vi "Handle_Plot.vi"(2 "Graph reference":refnum<vi>[](array[refnum]), 3 "System Monitor Variables (in)":T2={"Time"=[], "LI1CH1"=[], "LI1CH2"=[], "LI2CH1"=[], "LI2CH2"=[], "LI3CH1"=[], "LI3CH2"=[], "Field"=[], "Temp"=[], "Temp 2"=[], "Temp 3"=[], "N_Level"=[], "H_Level"=[], "Heat_370"=[], "Sorb_Heat"=[], "Still_Heat"=[], "Capacity"=[], "Loss"=[], "Magnet_Temperature"=[], "Lam_Pressure"=[], "Lam_NValve"=[], "370-T1"=[], "370-T2"=[], "370-T3"=[], "370-T4"=[], "370-T5"=[], "370-R1"=[], "370-R2"=[], "370-R3"=[], "370-R4"=[], "370-R5"=[], "372-T1"=[], "372-T2"=[], "372-T3"=[], "372-T4"=[], "372-T5"=[], "372-T6"=[], "372-R1"=[], "372-R2"=[], "372-R3"=[], "372-R4"=[], "372-R5"=[], "372-R6"=[], "Nada"=[nan], "K2440_Res"=[], "K2440_Current"=[], "VTI_Heater"=[], "VTI_NValve"=[], "LS340_Heater"=[], "K6221_Amplitude"=[], "K6221_Frequency"=[], "Cond_Pressure"=[], "Still_Pressure"=[], "FP_Out_Pressure"=[], "Dump_Pressure"=[], "V1"=[], "V2"=[], "V4"=[], "V5"=[], "V9"=[], "Forepump"=[], "Compressor"=[], "K6221_Offset"=[], "BoxTemp"=[], "By"=[], "Bz"=[], "Phi"=[], "heater-recond (%)"=[], "Dewar Pressure "=[], "JT-SP-Control"=[], "350 T1"=[], "350 T2"=[], "350 T3"=[], "350 T4"=[], "350 R1"=[], "350 R2"=[], "350 R3"=[], "350 R4"=[], "Angle"=[]}, 4 "Plot Array (in)":T1[](array[typedef]) {"Y-Axis Array" items=["Time", "LI1CH1", "LI1CH2", "LI2CH1", "LI2CH2", "LI3CH1", "LI3CH2", "Field", "Temp", "Temp 2", "Temp 3", "N_Level", "H_Level", "Heat_370", "Sorb_Heat", "Still_Heat", "Capacity", "Loss", "Magnet_Temperature", "Lam_Pressure", "Lam_NValve", "370-T1", "370-T2", "370-T3", "370-T4", "370-T5", "370-R1", "370-R2", "370-R3", "370-R4", "370-R5", "372-T1", "372-T2", "372-T3", "372-T4", "372-T5", "372-T6", "372-R1", "372-R2", "372-R3", "372-R4", "372-R5", "372-R6", "Nada", "K2440_Res", "K2440_Current", "VTI_Heater", "VTI_NValve", "LS340_Heater", "K6221_Amplitude", "K6221_Frequency", "Cond_Pressure", "Still_Pressure", "FP_Out_Pressure", "Dump_Pressure", "V1", "V2", "V4", "V5", "V9", "Forepump", "Compressor", "K6221_Offset", "BoxTemp", "By", "Bz", "Phi", "heater-recond (%)", "Dewar Pressure ", "JT-SP-Control", "350 T1", "350 T2", "350 T3", "350 T4", "350 R1", "350 R2", "350 R3", "350 R4", "Angle"]; "X-Axis" items=["Time", "LI1CH1", "LI1CH2", "LI2CH1", "LI2CH2", "LI3CH1", "LI3CH2", "Field", "Temp", "Temp 2", "Temp 3", "N_Level", "H_Level", "Heat_370", "Sorb_Heat", "Still_Heat", "Capacity", "Loss", "Magnet_Temperature", "Lam_Pressure", "Lam_NValve", "370-T1", "370-T2", "370-T3", "370-T4", "370-T5", "370-R1", "370-R2", "370-R3", "370-R4", "370-R5", "372-T1", "372-T2", "372-T3", "372-T4", "372-T5", "372-T6", "372-R1", "372-R2", "372-R3", "372-R4", "372-R5", "372-R6", "Nada", "K2440_Res", "K2440_Current", "VTI_Heater", "VTI_NValve", "LS340_Heater", "K6221_Amplitude", "K6221_Frequency", "Cond_Pressure", "Still_Pressure", "FP_Out_Pressure", "Dump_Pressure", "V1", "V2", "V4", "V5", "V9", "Forepump", "Compressor", "K6221_Offset", "BoxTemp", "By", "Bz", "Phi", "heater-recond (%)", "Dewar Pressure ", "JT-SP-Control", "350 T1", "350 T2", "350 T3", "350 T4", "350 R1", "350 R2", "350 R3", "350 R4", "Angle"]}) -> (1 "Measurement Graphs":T1[](array[typedef]) {"Y-Axis Array" items=["Time", "LI1CH1", "LI1CH2", "LI2CH1", "LI2CH2", "LI3CH1", "LI3CH2", "Field", "Temp", "Temp 2", "Temp 3", "N_Level", "H_Level", "Heat_370", "Sorb_Heat", "Still_Heat", "Capacity", "Loss", "Magnet_Temperature", "Lam_Pressure", "Lam_NValve", "370-T1", "370-T2", "370-T3", "370-T4", "370-T5", "370-R1", "370-R2", "370-R3", "370-R4", "370-R5", "372-T1", "372-T2", "372-T3", "372-T4", "372-T5", "372-T6", "372-R1", "372-R2", "372-R3", "372-R4", "372-R5", "372-R6", "Nada", "K2440_Res", "K2440_Current", "VTI_Heater", "VTI_NValve", "LS340_Heater", "K6221_Amplitude", "K6221_Frequency", "Cond_Pressure", "Still_Pressure", "FP_Out_Pressure", "Dump_Pressure", "V1", "V2", "V4", "V5", "V9", "Forepump", "Compressor", "K6221_Offset", "BoxTemp", "By", "Bz", "Phi", "heater-recond (%)", "Dewar Pressure ", "JT-SP-Control", "350 T1", "350 T2", "350 T3", "350 T4", "350 R1", "350 R2", "350 R3", "350 R4", "Angle"]; "X-Axis" items=["Time", "LI1CH1", "LI1CH2", "LI2CH1", "LI2CH2", "LI3CH1", "LI3CH2", "Field", "Temp", "Temp 2", "Temp 3", "N_Level", "H_Level", "Heat_370", "Sorb_Heat", "Still_Heat", "Capacity", "Loss", "Magnet_Temperature", "Lam_Pressure", "Lam_NValve", "370-T1", "370-T2", "370-T3", "370-T4", "370-T5", "370-R1", "370-R2", "370-R3", "370-R4", "370-R5", "372-T1", "372-T2", "372-T3", "372-T4", "372-T5", "372-T6", "372-R1", "372-R2", "372-R3", "372-R4", "372-R5", "372-R6", "Nada", "K2440_Res", "K2440_Current", "VTI_Heater", "VTI_NValve", "LS340_Heater", "K6221_Amplitude", "K6221_Frequency", "Cond_Pressure", "Still_Pressure", "FP_Out_Pressure", "Dump_Pressure", "V1", "V2", "V4", "V5", "V9", "Forepump", "Compressor", "K6221_Offset", "BoxTemp", "By", "Bz", "Phi", "heater-recond (%)", "Dewar Pressure ", "JT-SP-Control", "350 T1", "350 T2", "350 T3", "350 T4", "350 R1", "350 R2", "350 R3", "350 R4", "Angle"]})   [LabVIEW 2016]
uses:
  Global/Global Variables/System Monitor Cluster.ctl
  Plot.ctl
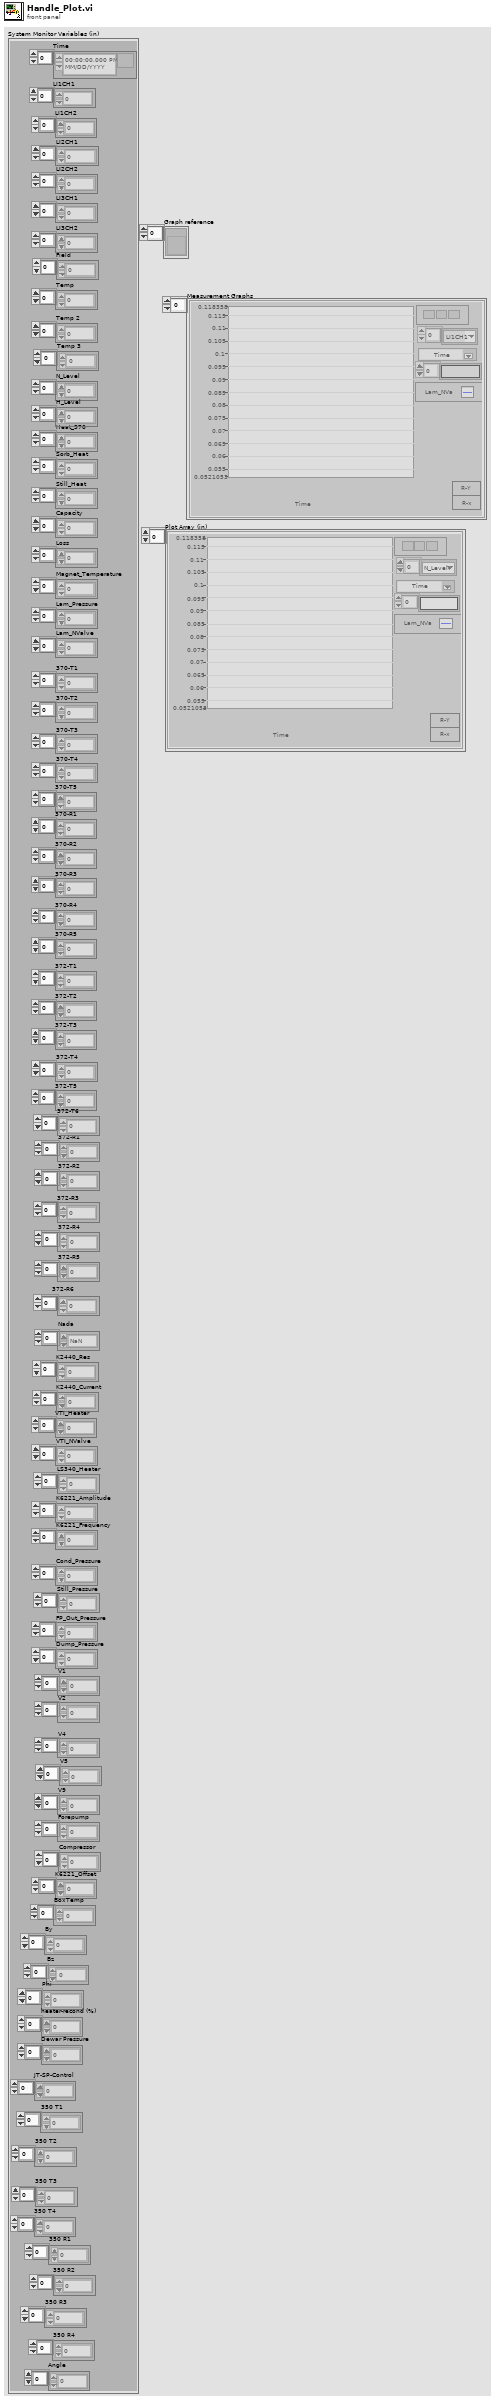
[diagram p1: front panel]
types:
  T1 = typedef "Plot.ctl" = cluster{"Measurement Graph":cluster{"Y":dbl[], "X":dbl[]}[], "X-Axis":i16, "Y-Axis Array":i16[], "Scale Plot":string[], "Rescale X":bool, "Rescale Y":bool}
  T2 = typedef "System Monitor Cluster.ctl" = cluster{"Time":timestamp[], "LI1CH1":dbl[], "LI1CH2":dbl[], "LI2CH1":dbl[], "LI2CH2":dbl[], "LI3CH1":dbl[], "LI3CH2":dbl[], "Field":dbl[], "Temp":dbl[], "Temp 2":dbl[], "Temp 3":dbl[], "N_Level":dbl[], "H_Level":dbl[], "Heat_370":dbl[], "Sorb_Heat":dbl[], "Still_Heat":dbl[], "Capacity":dbl[], "Loss":dbl[], "Magnet_Temperature":dbl[], "Lam_Pressure":dbl[], "Lam_NValve":dbl[], "370-T1":dbl[], "370-T2":dbl[], "370-T3":dbl[], "370-T4":dbl[], "370-T5":dbl[], "370-R1":dbl[], "370-R2":dbl[], "370-R3":dbl[], "370-R4":dbl[], "370-R5":dbl[], "372-T1":dbl[], "372-T2":dbl[], "372-T3":dbl[], "372-T4":dbl[], "372-T5":dbl[], "372-T6":dbl[], "372-R1":dbl[], "372-R2":dbl[], "372-R3":dbl[], "372-R4":dbl[], "372-R5":dbl[], "372-R6":dbl[], "Nada":dbl[], "K2440_Res":dbl[], "K2440_Current":dbl[], "VTI_Heater":dbl[], "VTI_NValve":dbl[], "LS340_Heater":dbl[], "K6221_Amplitude":dbl[], "K6221_Frequency":dbl[], "Cond_Pressure":dbl[], "Still_Pressure":dbl[], "FP_Out_Pressure":dbl[], "Dump_Pressure":dbl[], "V1":dbl[], "V2":dbl[], "V4":dbl[], "V5":dbl[], "V9":dbl[], "Forepump":dbl[], "Compressor":dbl[], "K6221_Offset":dbl[], "BoxTemp":dbl[], "By":dbl[], "Bz":dbl[], "Phi":dbl[], "heater-recond (%)":dbl[], "Dewar Pressure ":dbl[], "JT-SP-Control":dbl[], "350 T1":dbl[], "350 T2":dbl[], "350 T3":dbl[], "350 T4":dbl[], "350 R1":dbl[], "350 R2":dbl[], "350 R3":dbl[], "350 R4":dbl[], "Angle":dbl[]}
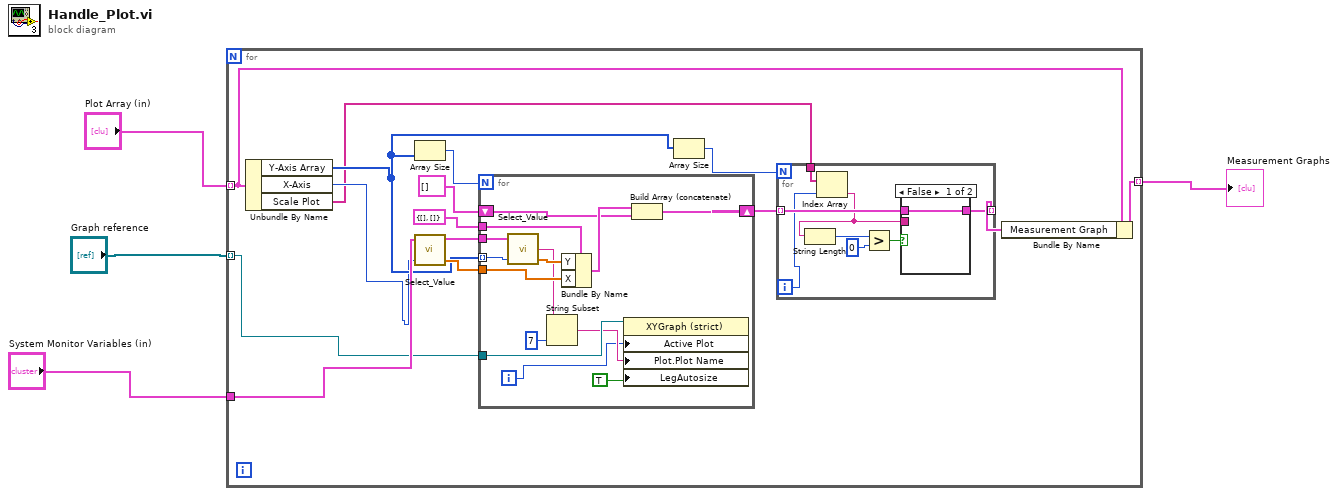
[diagram p0: block diagram]
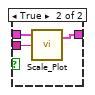
[diagram p2: hidden frame]
diagram:
  n1 = for {
    tunnel: "System Monitor Variables (in)" -> [w13]
    tunnel: [w7] -> w2 mode=indexing
    tunnel: "Plot Array (in)" -> [w9] mode=indexing
    tunnel: "Graph reference" -> [w5] mode=indexing
    n2 = Unbundle By Name(w9) -> ("Y-Axis Array"=w11:i16[], "X-Axis"=w10:i16, "Scale Plot"=w6:string[])
    n3 = Array Size(array=w11) -> (size(s)=w12:i32)
    n4 = call "Select_Value.vi"("Numerisch"=w10, "System Monitor Variables"=w13) -> ("Array"=w16:dbl[])  [unwired: 1 in, 2 out]
    n5 = for {
      N: w12 -> [_]
      tunnel: cluster{"X":dbl[], "Y":dbl[]} {"X"=[], "Y"=[]} -> [w44]
      tunnel: w11 -> [w42] mode=indexing
      tunnel: w13 -> [w41]
      shift-right: [w40] -> w14
      shift-left: cluster{"X":dbl[], "Y":dbl[]}[] [] -> [w33]
      tunnel: w16 -> [w39]
      tunnel: w5 -> [w36]
      i -> [w31]
      n6 = call "Select_Value.vi"("Numerisch"=w42, "System Monitor Variables"=w41) -> ("Array"=w43:dbl[], "String"=w37:string)  [unwired: 1 in, 1 out]
      n7 = String Subset(string=w37, length (rest)=7 ("length (rest)")) -> (substring=w32:string)  [unwired: 1 in]
      n8 = Bundle By Name(cluster=w44, "Y"=w43, "X"=w39) -> (w34:cluster{"X":dbl[], "Y":dbl[]})
      n9 = property on="Property Node" class="XYGraph (strict)"(reference=w36, "Active Plot"=w31, "Plot.Plot Name"=w32, "LegAutosize"=TRUE) -> ()  [unwired: 1 in, 2 out]
      n10 = Build Array (concatenate)(w34, w33) -> (w40:cluster{"X":dbl[], "Y":dbl[]}[])
    }
    n11 = Array Size(array=w11) -> (size(s)=w15:i32)
    n12 = for {
      N: w15 -> [_]
      tunnel: w14 -> [w25] mode=indexing
      tunnel: [w24] -> w8 mode=indexing
      tunnel: w6 -> [w21]
      i -> [w22]
      n13 = Index Array(array=w21, index=w22) -> (element=w20:string)
      n14 = String Length(string=w20) -> (length=w23:i32)
      n15 = Greater?(x=w23, y=0) -> (0:w19:bool)
      n16 = case shown="False" w19 {
        tunnel: w25 -> [w27 w30]
        tunnel: [w27 w29] -> w24
        tunnel: w20 -> [_ w28]
        frame False {
        }
        frame True {
          n17 = call "Scale_Plot.vi"("Cluster"=w30, "String"=w28) -> ("Cluster 2"=w29:cluster{"Y":dbl[], "X":dbl[]})  [unwired: 4 in]
        }
      }
    }
    n18 = Bundle By Name(cluster=w9, "Measurement Graph"=w8) -> (w7:T1)
  }
  "Measurement Graphs" <- w2
